vi "WfmDataAccessor WriteData.vi"(8 "error in (no error)":errorcluster, 9 "XML":string, 10 "WfmData":u64[](array[numeric]), 11 "WfmDataAccessor in":refnum<class "WfmDataAccessor.lvclass">) -> (0 "error out":errorcluster, 3 "WfmDataAccessor out":refnum<class "WfmDataAccessor.lvclass">)   [LabVIEW 2018, in "WfmDataAccessor.lvclass"]
uses:
  WfmDataAccessor.lvclass
  WfmDataAccessor.lvclass/WfmDataAccessor.ctl
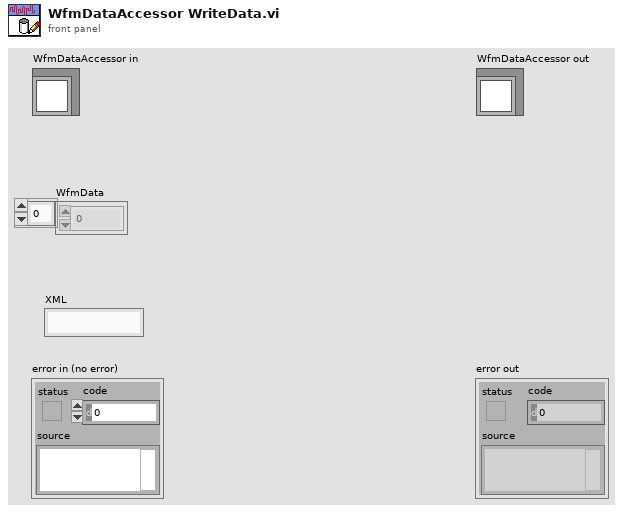
[diagram p1: front panel]
types:
  T1 = enum16{"open", "replace", "create", "open or create", "replace or create", "replace or create with confirmation"}
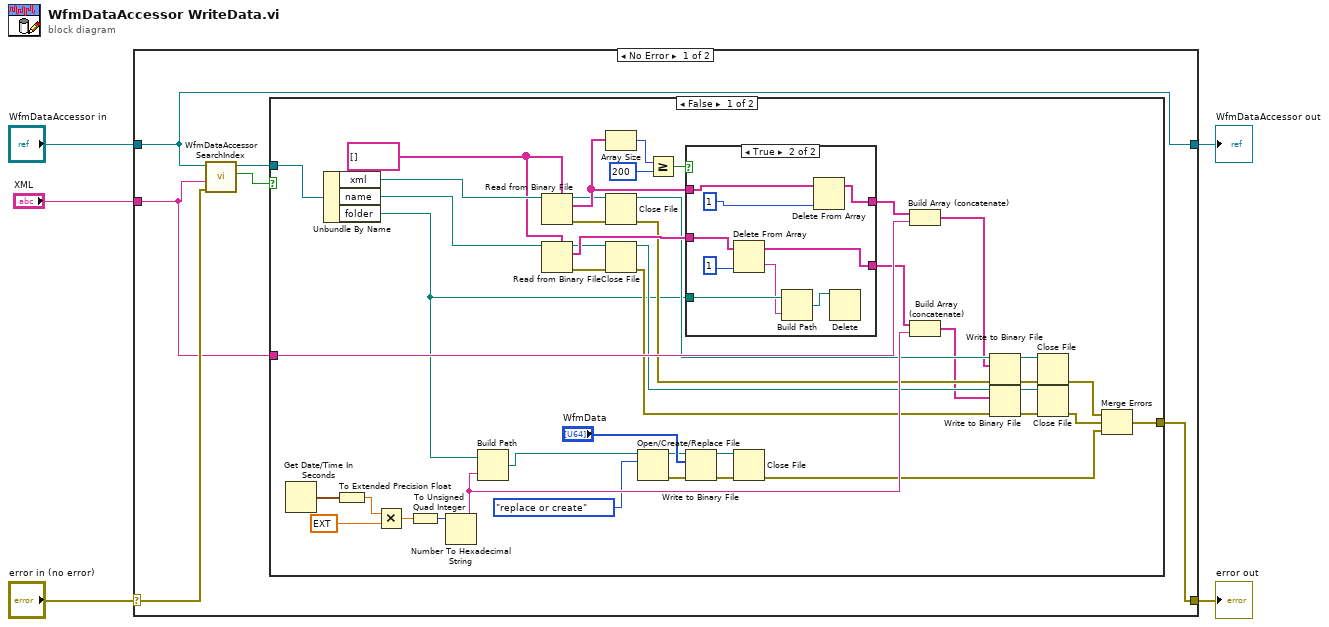
[diagram p0: block diagram]
diagram:
  n1 = case shown="No Error" "error in (no error)" {
    selector: "error in (no error)" -> [w11 w68]
    tunnel: [w7 w68] -> w4
    tunnel: [w6 w67] -> w2
    tunnel: "WfmDataAccessor in" -> [w6 w67]
    tunnel: "XML" -> [w8 _]
    frame No Error {
      n2 = call-dynamic "WfmDataAccessor SearchIndex.vi"("error in (no error)"=w11, "XML in"=w8, "WfmDataAccessor in"=w6) -> ("Found"=w10:bool, "WfmDataAccessor out"=w9:refnum<class "WfmDataAccessor.lvclass">)  [unwired: 5 in, 2 out]
      n3 = case shown="False" w10 {
        tunnel: w9 -> [w51 _]
        tunnel: w8 -> [w32 _]
        tunnel: [w21 _] -> w7
        frame False {
          w43 = string[] []
          n4 = Get Date/Time In Seconds() -> (seconds since 1Jan1904=w50:timestamp)
          n5 = Unbundle By Name(w51) -> ("xml"=w44:path, "name"=w45:path, "folder"=w23:path)
          n6 = To Extended Precision Float(1:w50) -> (0:w49:ext)
          n7 = Multiply(x=w49, y=ext 100.0) -> (x*y=w47:ext)
          n8 = To Unsigned Quad Integer(1:w47) -> (0:w46:u64)
          n9 = Number To Hexadecimal String(2:w46) -> (0:w30:string)  [unwired: 1 in]
          n10 = Build Path(base path=w23, name or relative path=w30) -> (appended path=w52:path)
          n11 = Read from Binary File(5:w43, 11:w44) -> (0:w36:errorcluster, 2:w39:string[], 3:w37:refnum<file>)  [unwired: 4 in, 1 out]
          n12 = Read from Binary File(5:w43, 11:w45) -> (0:w34:errorcluster, 2:w38:string[], 3:w35:refnum<file>)  [unwired: 4 in, 1 out]
          n13 = Array Size(array=w39) -> (size(s)=w42:i32)
          n14 = Close File(refnum=w37, error in=w36) -> (path=w26:path, error out=w29:errorcluster)
          n15 = Close File(refnum=w35, error in=w34) -> (path=w27:path, error out=w28:errorcluster)
          n16 = Open/Create/Replace File(file path (use dialog)=w52, operation (0:open)=T1."replace or create") -> (refnum out=w14:refnum<file>, error out=w13:errorcluster)  [unwired: 4 in, 1 out]
          n17 = Greater Or Equal?(x=w42, y=200) -> (x >= y?=w40:bool)
          n18 = case shown="True" w40 {
            tunnel: w39 -> [w57 w66]
            tunnel: w38 -> [w56 w62]
            tunnel: [w57 w64] -> w33
            tunnel: [w56 w63] -> w31
            tunnel: w23 -> [_ w60]
            frame False {
            }
            frame True {
              n19 = Delete From Array(array=w62, index=1) -> (deleted portion=w59:string, array with subset deleted=w63:string[])  [unwired: 1 in]
              n20 = Build Path(base path=w60, name or relative path=w59) -> (appended path=w58:path)
              n21 = Delete From Array(array=w66, index=1) -> (array with subset deleted=w64:string[])  [unwired: 1 in, 1 out]
              n22 = Delete(path (use dialog)=w58) -> ()  [unwired: 4 in, 3 out]
            }
          }
          n23 = Write to Binary File(file (use dialog)=w14, data="WfmData", error in=w13) -> (refnum out=w55:refnum<file>, error out=w54:errorcluster)  [unwired: 3 in, 1 out]
          n24 = Close File(refnum=w55, error in=w54) -> (error out=w22:errorcluster)  [unwired: 1 out]
          n25 = Build Array (concatenate)(w33, w32) -> (w24:string[])
          n26 = Build Array (concatenate)(w31, w30) -> (w25:string[])
          n27 = Write to Binary File(file (use dialog)=w26, data=w24, error in=w29) -> (refnum out=w19:refnum<file>, error out=w20:errorcluster)  [unwired: 3 in, 1 out]
          n28 = Write to Binary File(file (use dialog)=w27, data=w25, error in=w28) -> (refnum out=w17:refnum<file>, error out=w16:errorcluster)  [unwired: 3 in, 1 out]
          n29 = Close File(refnum=w19, error in=w20) -> (error out=w18:errorcluster)  [unwired: 1 out]
          n30 = Close File(refnum=w17, error in=w16) -> (error out=w15:errorcluster)  [unwired: 1 out]
          n31 = Merge Errors(w18, w15, w22) -> (w21:errorcluster)
        }
        frame True {
        }
      }
    }
    frame Error {
    }
  }
  "error out" <- w4
  "WfmDataAccessor out" <- w2
